vi "Agilent VNA Set Channel.vi"(7 "Agilent VNA":T1, 8 "error in (no error)":errorcluster, 10 "Channel":i8=1 min=1 max=99 step=1, 11 "VISA Resource Name":refnum<visa-resource-name>) -> (0 "error out":errorcluster, 3 "dup VISA Resource Name":refnum<visa-resource-name>)   [LabVIEW 2011]
uses:
  TypeDefs/Agilent VNA Instrument Info.ctl
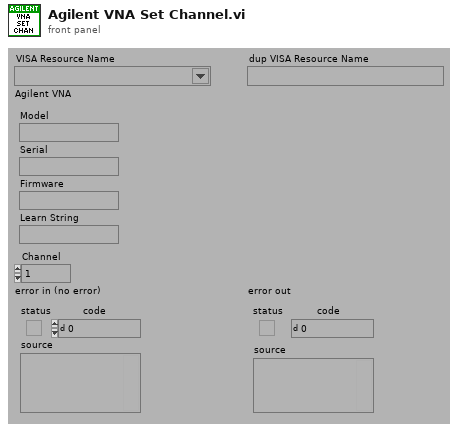
[diagram p1: front panel]
types:
  T1 = typedef "Agilent VNA Instrument Info.ctl" = cluster{"Model":string, "Serial":string, "Firmware":string, "Learn String":string}
  T2 = typedef "Agilent VNA Model.ctl" = enum16{"Not Supported", "8510X", "8719X", "8720X", "8722X", "8753X", "ENA", "PNA", "Field Fox"}
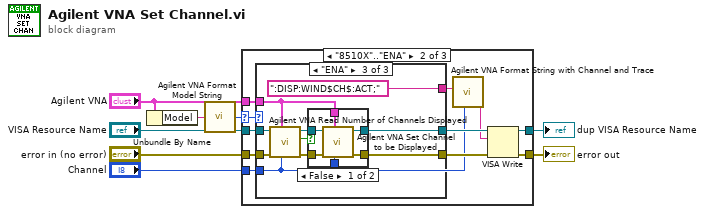
[diagram p0: block diagram]
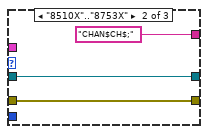
[diagram p4: hidden frame]
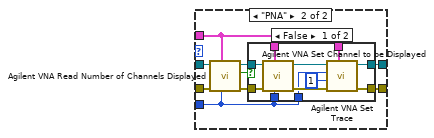
[diagram p7: hidden frame]
diagram:
  n1 = Unbundle By Name("Agilent VNA") -> ("Model"=w2:string)
  n2 = call "Agilent VNA Format Model String.vi"("Model"=w2) -> ("Model"=w3:T2)
  n3 = case shown="\"8510X\"..\"ENA\"" w3 {
    selector: w3 -> [_ w11 w47]
    tunnel: [w10 w21 w45] -> w8
    tunnel: [w9 w20 w46] -> w7
    tunnel: "VISA Resource Name" -> [w10 w19 w51]
    tunnel: "error in (no error)" -> [w9 w18 w50]
    tunnel: "Agilent VNA" -> [_ w15 w49]
    tunnel: "Channel" -> [_ w12 w48]
    frame "Not Supported", "Field Fox" {
      # "Field Fox only has one channel."
    }
    frame "8510X".."ENA" {
      n4 = case shown="\"ENA\"" w11 {
        tunnel: [_ "CHAN$CH$;" ":DISP:WIND$CH$:ACT;"] -> w13
        tunnel: w19 -> [w23 w25 w35]
        tunnel: w18 -> [w22 w24 w36]
        tunnel: [w23 w25 w27] -> w17
        tunnel: [w22 w24 w28] -> w16
        tunnel: w15 -> [_ _ w31]
        tunnel: w12 -> [_ _ w30]
        frame "Not Supported", "PNA", "Field Fox" {
        }
        frame "8510X".."8753X" {
        }
        frame "ENA" {
          n5 = call "Agilent VNA Read Number of Channels Displayed.vi"("Channel to be Displayed"=w30, "Agilent VNA"=w31, "error in (no error)"=w36, "VISA Resource Name"=w35) -> ("error out"=w32:errorcluster, "Displayed?"=w34:bool, "dup VISA Resource Name"=w33:refnum<visa-resource-name>)  [unwired: 5 out]
          n6 = case shown="False" w34 {
            tunnel: w33 -> [w39 w43]
            tunnel: w32 -> [w42 w44]
            tunnel: [w41 w44] -> w28
            tunnel: [w40 w43] -> w27
            tunnel: w30 -> [w38 _]
            tunnel: w31 -> [w37 _]
            frame False {
              n7 = call "Agilent VNA Set Channel to be Displayed.vi"("Channel to be Displayed"=w38, "Agilent VNA"=w37, "error in (no error)"=w42, "VISA Resource Name"=w39) -> ("error out"=w41:errorcluster, "dup VISA Resource Name"=w40:refnum<visa-resource-name>)  [unwired: 6 out]
            }
            frame True {
            }
          }
        }
      }
      n8 = call "Agilent VNA Format String with Channel and Trace.vi"("Channel"=w12, "String"=w13) -> ("String Out"=w14:string)  [unwired: 1 in, 6 out]
      n9 = VISA Write(VISA resource name=w17, write buffer=w14, error in (no error)=w16) -> (VISA resource name out=w21:refnum<visa-resource-name>, error out=w20:errorcluster)  [unwired: 1 out]
    }
    frame "PNA" {
      n10 = case shown="\"Not Supported\"..\"ENA\", \"Field Fox\"" w47 {
        tunnel: w51 -> [w53 w58]
        tunnel: w50 -> [w52 w59]
        tunnel: [w53 w57] -> w45
        tunnel: [w52 w56] -> w46
        tunnel: w49 -> [_ w55]
        tunnel: w48 -> [_ w54]
        frame "Not Supported".."ENA", "Field Fox" {
        }
        frame "PNA" {
          n11 = call "Agilent VNA Read Number of Channels Displayed.vi"("Channel to be Displayed"=w54, "Agilent VNA"=w55, "error in (no error)"=w59, "VISA Resource Name"=w58) -> ("error out"=w60:errorcluster, "Displayed?"=w62:bool, "dup VISA Resource Name"=w61:refnum<visa-resource-name>)  [unwired: 5 out]
          n12 = case shown="False" w62 {
            tunnel: w61 -> [w72 w74]
            tunnel: w60 -> [w73 w75]
            tunnel: [w66 w75] -> w56
            tunnel: [w68 w74] -> w57
            tunnel: w54 -> [w71 _]
            tunnel: w55 -> [w70 _]
            tunnel: w55 -> [w65 _]
            tunnel: w54 -> [w64 _]
            frame False {
              n13 = call "Agilent VNA Set Channel to be Displayed.vi"("Channel to be Displayed"=w71, "Agilent VNA"=w70, "error in (no error)"=w73, "VISA Resource Name"=w72) -> ("error out"=w67:errorcluster, "dup VISA Resource Name"=w69:refnum<visa-resource-name>)  [unwired: 6 out]
              n14 = call "Agilent VNA Set Trace.vi"("Agilent VNA"=w65, "error in (no error)"=w67, "Trace"=i8 1, "Channel"=w64, "VISA Resource Name"=w69) -> ("error out"=w66:errorcluster, "dup VISA Resource Name"=w68:refnum<visa-resource-name>)  [unwired: 5 out]
            }
            frame True {
            }
          }
        }
      }
    }
  }
  "dup VISA Resource Name" <- w8
  "error out" <- w7
